vi "Add to Tree (Internal).vi"(6 "Display Text Override":string, 7 "Add children? (F)":bool, 8 "error in (no error)":errorcluster, 9 "Parent Tag":string, 10 "Tree Manager in":refnum<class "Tree Manager.lvclass">, 11 "Data Item in":refnum<class "Data Item.lvclass">) -> (0 "error out":errorcluster, 1 "New Tag":string, 2 "Tree Manager out":refnum<class "Tree Manager.lvclass">, 3 "Data Item out":refnum<class "Data Item.lvclass">)   [LabVIEW 2023, in "VILab.lvlib" / "Data Item.lvclass"]
uses:
  Data Item.lvclass
  Tree Manager/Tree Manager.lvclass
  Data Item.lvclass/Data Item.ctl
panel:
  in  "Child only? (F)":bool
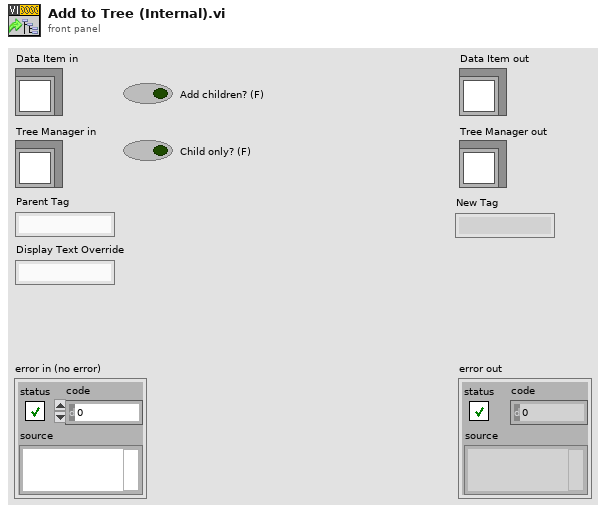
[diagram p1: front panel]
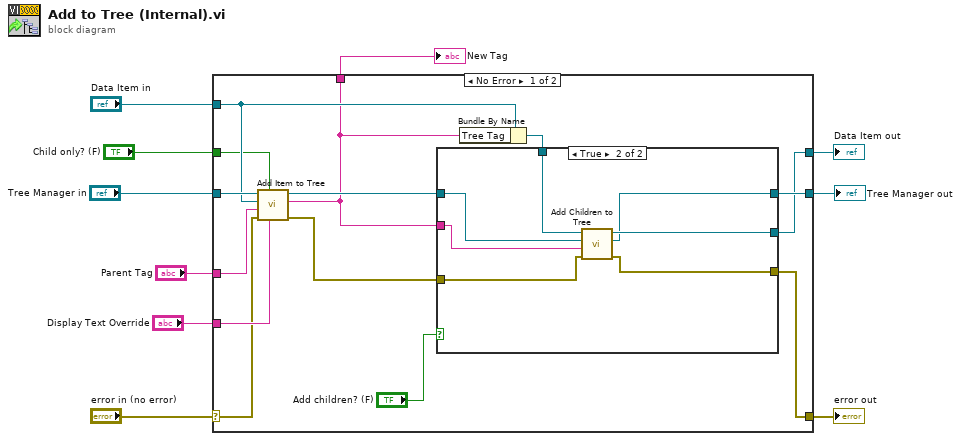
[diagram p0: block diagram]
diagram:
  n1 = case shown="No Error" "error in (no error)" {
    selector: "error in (no error)" -> [w13 w37]
    tunnel: [w17 w37] -> w9
    tunnel: [w18 w36] -> w7
    tunnel: "Data Item in" -> [w14 w36]
    tunnel: "Tree Manager in" -> [w24 w35]
    tunnel: "Parent Tag" -> [w23 _]
    tunnel: [w20 w35] -> w4
    tunnel: "Display Text Override" -> [w15 _]
    tunnel: [w12 _] -> w2
    tunnel: "Child only? (F)" -> [w11 _]
    frame No Error {
      n2 = call "Add Item to Tree.vi"("Display Text Override"=w15, "Child only? (F)"=w11, "error in (no error)"=w13, "Parent Tag"=w23, "Data Item"=w14, "Tree Manager in"=w24) -> ("error out"=w21:errorcluster, "New Tag"=w12:string, "Tree Manager out"=w22:refnum<class "Tree Manager.lvclass">)  [unwired: 3 in]
      n3 = Bundle By Name(cluster=w14, "Tree Tag"=w12) -> (w19:refnum<class "Data Item.lvclass">)
      n4 = case shown="True" "Add children? (F)" {
        tunnel: w22 -> [w26 w34]
        tunnel: w21 -> [w25 w32]
        tunnel: w12 -> [_ w33]
        tunnel: [w26 w30] -> w20
        tunnel: w19 -> [w27 w28]
        tunnel: [w27 w31] -> w18
        tunnel: [w25 w29] -> w17
        frame False {
        }
        frame True {
          n5 = call "Add Children to Tree.vi"("error in (no error)"=w32, "Parent Tag"=w33, "Tree Manager in"=w34, "Data Item in"=w28) -> ("error out"=w29:errorcluster, "Tree Manager out"=w30:refnum<class "Tree Manager.lvclass">, "Data Item out"=w31:refnum<class "Data Item.lvclass">)  [unwired: 5 in]
        }
      }
    }
    frame Error {
    }
  }
  "error out" <- w9
  "Data Item out" <- w7
  "Tree Manager out" <- w4
  "New Tag" <- w2
